vi "Read Drop_out.vi"(8 "error in (no error)":errorcluster, 11 "Solenoid in":refnum<class "Solenoid.lvclass">) -> (0 "error out":errorcluster, 2 "Drop_out":T1={"V"=24.0, "I"=0.5, "V_reduced"=4.0, "V_perturb"=0.01, "Plunger_Threshold"=0.01}, 3 "Solenoid out":refnum<class "Solenoid.lvclass">)   [LabVIEW 2025, in "Solenoid.lvclass"]
uses:
  Solenoid.lvclass
  Solenoid.lvclass/Solenoid.ctl
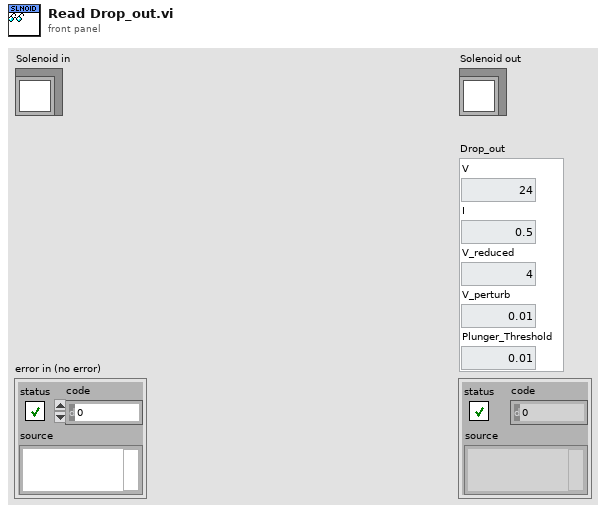
[diagram p1: front panel]
types:
  T1 = cluster{"V":dbl, "I":dbl, "V_reduced":dbl, "V_perturb":dbl, "Plunger_Threshold":dbl}
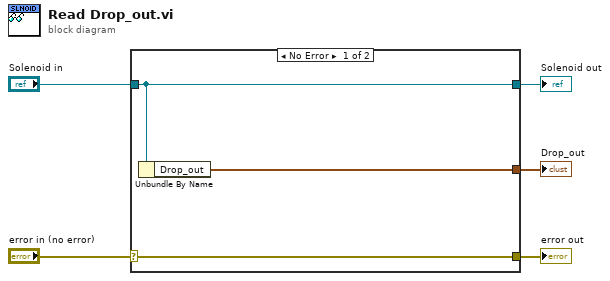
[diagram p0: block diagram]
diagram:
  n1 = case shown="No Error" "error in (no error)" {
    selector: "error in (no error)" -> [w8 w9]
    tunnel: [w8 w9] -> w4
    tunnel: [w7 w10] -> w2
    tunnel: "Solenoid in" -> [w7 w10]
    tunnel: [w6 _] -> w1
    frame No Error {
      n2 = Unbundle By Name(w7) -> ("Drop_out"=w6:T1)
    }
    frame Error {
    }
  }
  "error out" <- w4
  "Solenoid out" <- w2
  "Drop_out" <- w1
